vi "HKinTDMS_ECD.vi"(1 "Methode":i32, 2 "error in (no error)":errorcluster, 3 "Kanäle":string[](array[string])) -> (0 "error out":errorcluster)   [LabVIEW 2017]
uses:
  GVMWHorst_ECD.vi
  GVHK1Hz_ECD.vi
  GVaktuelleTDMS_ECD.vi
  GVZeitenZyklen_ECD.vi
  GVProbenvol_ECD.vi
  GVVentilposition_ECD.vi
  GVUTC_ECD.vi
  <vilib>/NI_Real-Time Target Support.lvlib
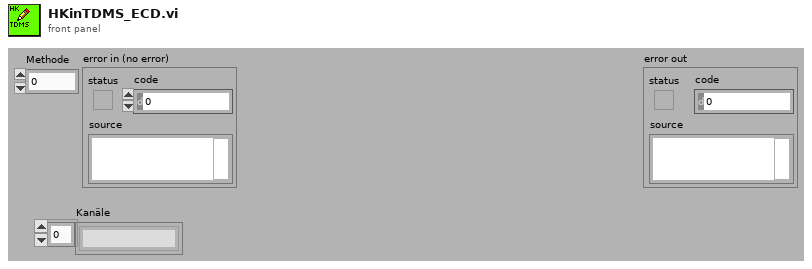
[diagram p1: front panel]
types:
  T1 = typedef "LVDateTimeRec.ctl" = cluster{"Sekundenbruchteil":dbl, "Sekunde":i32, "Minute":i32, "Stunde":i32, "Tag des Monats":i32, "Monat":i32, "Jahr":i32, "Wochentag":i32, "Tag des Jahres":i32, "DST":i32}
  T2 = typedef "NI_Real-Time Target Support.lvlib/RT CPU Load.ctl" = cluster{"Total (%)":dbl, "Time Critical (%)":dbl, "Timed Structures (%)":dbl, "High (%)":dbl, "Above Normal (%)":dbl, "Normal (%)":dbl, "Background (%)":dbl, "Idle (%)":dbl, "ISR (%)":dbl}
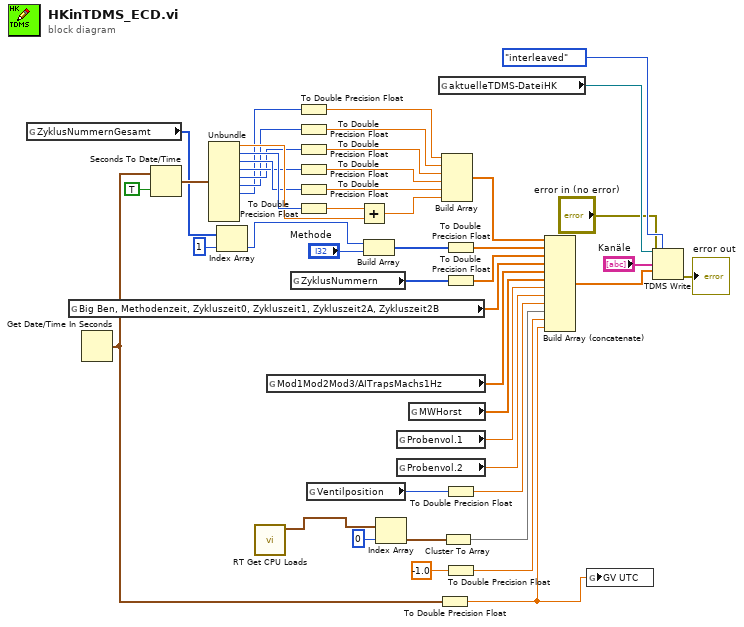
[diagram p0: block diagram]
diagram:
  n1 = global read "GVZeitenZyklen_ECD.vi" "ZyklusNummernGesamt"() -> (w36:i32[])
  n2 = global read "GVZeitenZyklen_ECD.vi" "Big Ben, Methodenzeit, Zykluszeit0, Zykluszeit1, Zykluszeit2A, Zykluszeit2B"() -> (w34:dbl[])
  n3 = Get Date/Time In Seconds() -> (seconds since 1Jan1904=w21:timestamp)
  n4 = Seconds To Date/Time(time stamp (now)=w21, to UTC (F)=TRUE ("in Weltzeit (F)")) -> (date time rec=w44:T1)
  n5 = Unbundle(w44) -> ("Sekundenbruchteil"=w18:dbl, "Sekunde"=w20:i32, "Minute"=w15:i32, "Stunde"=w13:i32, "Tag des Monats"=w11:i32, "Monat"=w9:i32, "Jahr"=w7:i32)  [unwired: 3 out]
  n6 = Index Array(array=w36, index=1 ("Index")) -> (element=w45:i32)
  n7 = call <vilib>:"RT Get CPU Loads.vi"() -> ("CPU loads"=w2:T2[])  [unwired: 10 in, 1 out]
  n8 = global read "GVHK1Hz_ECD.vi" "Mod1Mod2Mod3/AITrapsMachs1Hz"() -> (w31:dbl[])
  n9 = global read "GVZeitenZyklen_ECD.vi" "ZyklusNummern"() -> (w35:i32[])
  n10 = To Double Precision Float(number=w7) -> (double precision float=w6:dbl)
  n11 = To Double Precision Float(number=w9) -> (double precision float=w8:dbl)
  n12 = To Double Precision Float(number=w11) -> (double precision float=w10:dbl)
  n13 = To Double Precision Float(number=w13) -> (double precision float=w12:dbl)
  n14 = To Double Precision Float(number=w15) -> (double precision float=w14:dbl)
  n15 = To Double Precision Float(number=w20) -> (double precision float=w19:dbl)
  n16 = global read "GVVentilposition_ECD.vi" "Ventilposition"() -> (w41:i32)
  n17 = Add(x=w19, y=w18) -> (x+y=w17:dbl)
  n18 = Build Array(w45, "Methode") -> (w46:i32[])
  n19 = Index Array(array=w2, index=0) -> (element=w22:T2)
  n20 = global read "GVProbenvol_ECD.vi" "Probenvol.1"() -> (w37:dbl)
  n21 = global read "GVProbenvol_ECD.vi" "Probenvol.2"() -> (w38:dbl)
  n22 = global read "GVMWHorst_ECD.vi" "MWHorst"() -> (w30:dbl[])
  n23 = global read "GVaktuelleTDMS_ECD.vi" "aktuelleTDMS-DateiHK"() -> (w32:refnum<k34>)
  n24 = To Double Precision Float(number=w21) -> (double precision float=w5:dbl)
  n25 = Build Array(w6, w8, w10, w12, w14, w17) -> (w16:dbl[])
  n26 = Cluster To Array(cluster=w22) -> (array=w24:dbl[])
  n27 = To Double Precision Float(number=w46) -> (double precision float=w28:dbl[])
  n28 = To Double Precision Float(number=w35) -> (double precision float=w29:dbl[])
  n29 = To Double Precision Float(number=w41) -> (double precision float=w42:dbl)
  n30 = To Double Precision Float(number=-1.0 ("Zahl")) -> (double precision float=w23:dbl)
  n31 = Build Array (concatenate)(w16, w28, w29, w34, w31, w30, w37, w38, w42, w24, w23, w5) -> (w39:dbl[])
  n32 = global write "GVUTC_ECD.vi" "GV UTC"(w5) -> ()
  n33 = TDMS Write(0:w32, 1:enum16{"decimated", "interleaved"}."interleaved" ("Daten-Layout (0:dezimiert)"), 7:"Kanäle", 9:w39, 11:"error in (no error)") -> (15:→"error out":errorcluster)  [unwired: 1 in, 3 out]
